vi "SPI Write Read.vi"(5 "CS Pin (10)":u8=10, 7 "SPI Frame Size":u8, 8 "Error In":errorcluster, 9 "Data":u8[](array[numeric]), 10 "SPI Channel (0)":u8, 11 "LINX Resource":T2) -> (0 "Error Out":errorcluster, 1 "Read Data":u8[](array[numeric]), 3 "LINX Resource":T2)   [LabVIEW 2013, in "LVH-LINX.lvlib"]
doc: "Write/Read the specified SPI channel. SPI is full duplex, therefore the write and read operations take place simultaneously."
uses:
  <vilib>/LabVIEW Hacker/LINX/LVH-LINX.lvlib
  <vilib>/LabVIEW Hacker/LINX/Private/Type Defs/LINX Ref.ctl
  <vilib>/LabVIEW Hacker/LINX/Private/Type Defs/Platform.ctl
  <vilib>/LabVIEW Hacker/LINX/Private/Type Defs/Interface.ctl
  <vilib>/LabVIEW Hacker/LINX/Private/Device/Type Defs/LINX Device Config.ctl
  <vilib>/LabVIEW Hacker/LINX/Private/Device/Type Defs/TCP Config.ctl
  <vilib>/LabVIEW Hacker/LINX/Private/Type Defs/Device Family.ctl
  <vilib>/LabVIEW Hacker/LINX/Private/Type Defs/Peripherals/SPI/SPI CS Logic Level.ctl
  <vilib>/LabVIEW Hacker/LINX/Private/Type Defs/Peripheral.ctl
  <vilib>/LabVIEW Hacker/LINX/Private/Type Defs/Channel FGV States.ctl
  <vilib>/LabVIEW Hacker/LINX/Private/Device/Device.lvlib
  <vilib>/myRIO/Common/Instrument Driver Framework/myRIO v1.0/SPI/typedefs/SPI Frame Length.ctl
  <vilib>/myRIO/Common/Instrument Driver Framework/myRIO v1.0/SPI/typedefs/SPI Data Direction.ctl
  <vilib>/myRIO/Common/Instrument Driver Framework/myRIO v1.0/SPI/typedefs/SPI Clock Polarity.ctl
  <vilib>/myRIO/Common/Instrument Driver Framework/myRIO v1.0/SPI/typedefs/SPI Clock Phase.ctl
  <vilib>/myRIO/Instrument Drivers/Onboard IO/SPI/typedefs/SPI Configuration.ctl
  <vilib>/myRIO/Common/Instrument Driver Framework/myRIO v1.0/SPI/typedefs/SPI Channels Enum.ctl
  <vilib>/myRIO/Common/Instrument Driver Framework/Utilities/typedefs/Generic FPGA Reference.ctl
  <vilib>/myRIO/Common/Instrument Driver Framework/Utilities/typedefs/myRIO v1.0 Reference.ctl
  <vilib>/myRIO/Common/Instrument Driver Framework/Utilities/typedefs/Hardware Version Enum.ctl
  <vilib>/myRIO/Common/Instrument Driver Framework/Utilities/typedefs/myRIO Generic Hardware Reference.ctl
  <vilib>/myRIO/Instrument Drivers/Onboard IO/SPI/typedefs/SPI Reference.ctl
panel:
  in  "CS Logic Level":T1
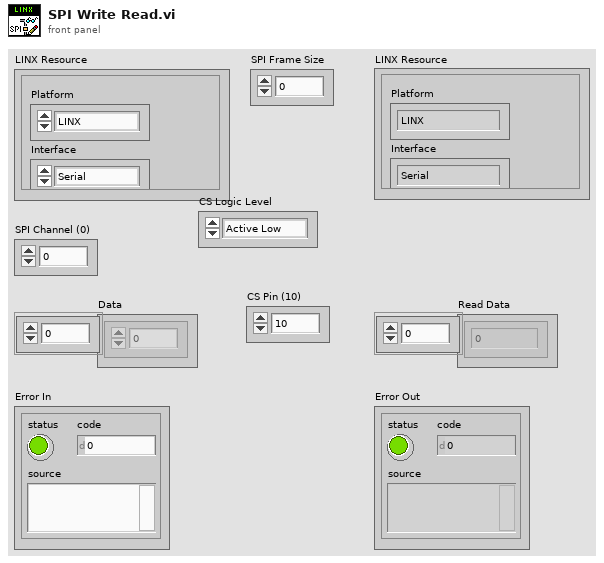
[diagram p1: front panel]
types:
  T1 = typedef "LVH-LINX.lvlib/SPI CS Logic Level.ctl" = enum8{"Active Low", "Active High"}
  T2 = typedef "LVH-LINX.lvlib/LINX Ref.ctl" = cluster{"Platform":T3, "Interface":T4, "LINX Device Config":T5}
  T3 = typedef "LVH-LINX.lvlib/Platform.ctl" = enum16{"LINX", "myRIO"}
  T4 = typedef "LVH-LINX.lvlib/Interface.ctl" = enum16{"Serial", "TCP"}
  T5 = typedef "LVH-LINX.lvlib/Device.lvlib/LINX Device Config.ctl" = cluster{"Interface":T4, "COM Port":refnum<visa-resource-name>, "TCP Configuration":T6, "Device Family":T7, "Device ID":u8, "Device Name":string, "TCP Ref":refnum<k5>}
  T6 = typedef "LVH-LINX.lvlib/Device.lvlib/TCP Config.ctl" = cluster{"IP Address":string, "Port":u16}
  T7 = typedef "LVH-LINX.lvlib/Device Family.ctl" = enum8{"National Instruments", "Digilent", "Arduino"}
  T8 = typedef "LVH-LINX.lvlib/Peripheral.ctl" = enum8{"DI", "DO", "AI", "AO", "PWM", "QE", "UART", "I2C", "SPI", "CAN"}
  T9 = typedef "LVH-LINX.lvlib/Channel FGV States.ctl" = enum16{"Initialize", "Get", "Set"}
  T10 = typedef "SPI.lvlib/SPI Reference.ctl" = cluster{"myRIO Reference":T11, "SPI Channels Enum":T15, "SPI Configuration":T16}
  T11 = typedef "myRIO Generic Hardware Reference.ctl" = cluster{"myRIO Model":T12, "myRIO Hardware Reference":T13}
  T12 = typedef "Hardware Version Enum.ctl" = enum16{"Unknown", "myRIO-1900", "myRIO-1950"}
  T13 = typedef "myRIO v1.0 Reference.ctl" = cluster{"Generic FPGA Reference":T14, "Allow multiple opens":bool}
  T14 = typedef "Generic FPGA Reference.ctl" = refnum<k20>
  T15 = typedef "SPI Channels Enum.ctl" = enum16{"Not Connected", "A/SPI", "B/SPI"}
  T16 = typedef "SPI.lvlib/SPI Configuration.ctl" = cluster{"Frequency (Hz)":dbl, "Clock Phase":T17, "Clock Polarity":T18, "Data Direction":T19, "Frame Length":T20}
  T17 = typedef "SPI Clock Phase.ctl" = enum8{"Leading", "Trailing"}
  T18 = typedef "SPI Clock Polarity.ctl" = enum8{"Low", "High"}
  T19 = typedef "SPI Data Direction.ctl" = enum8{"Most Significant Bit First", "Least Significant Bit First"}
  T20 = typedef "SPI Frame Length.ctl" = u8
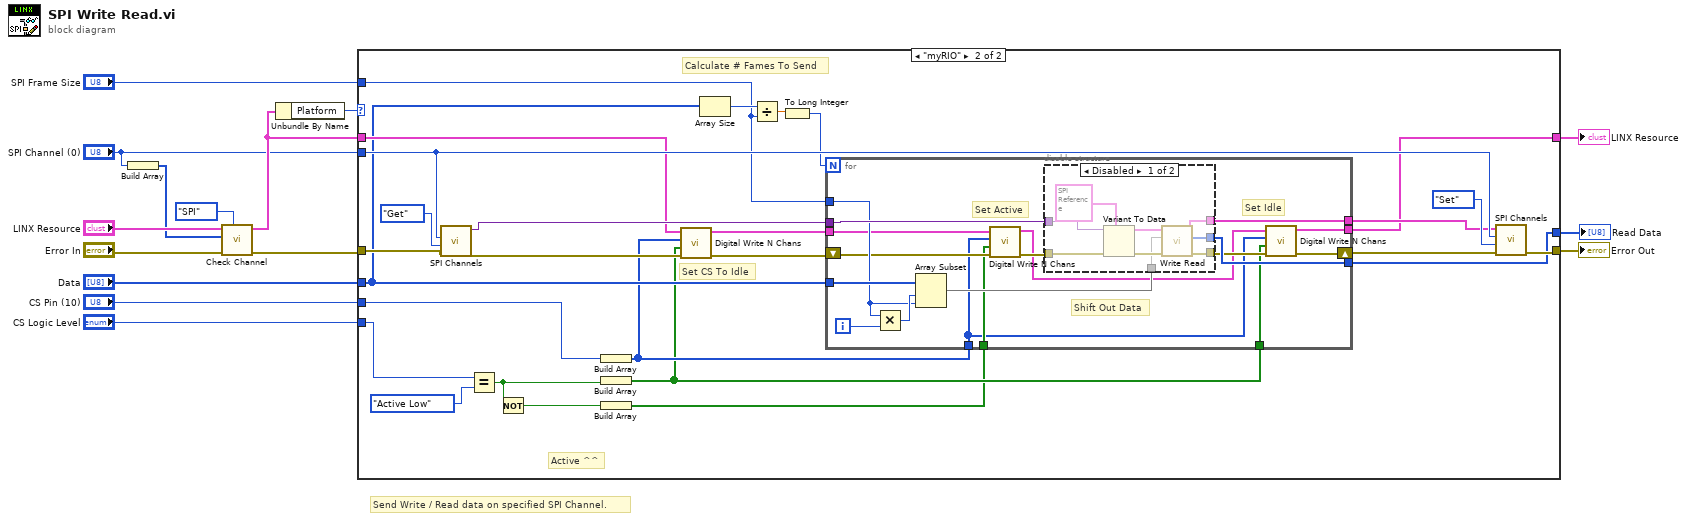
[diagram p0: block diagram]
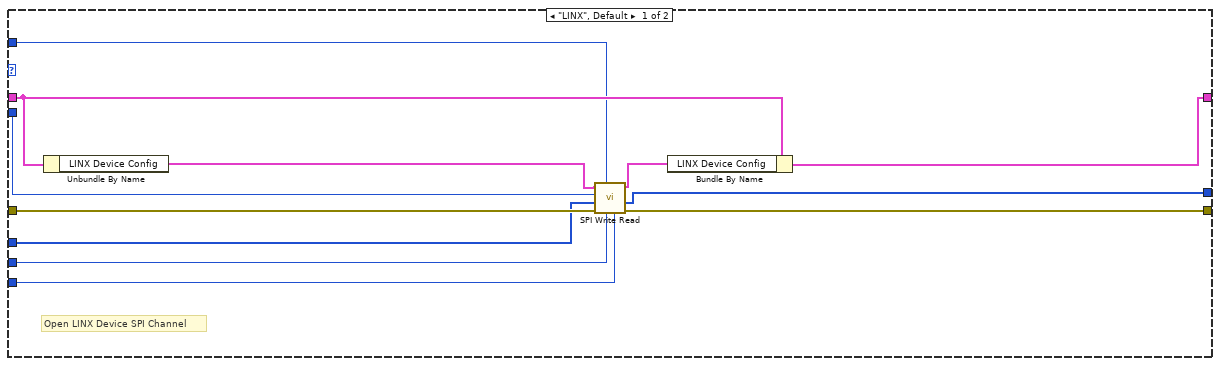
[diagram p2: hidden frame]
diagram:
  # "Send Write / Read data on specified SPI Channel."
  n1 = Build Array("SPI Channel (0)") -> (w9:u8[])
  n2 = call <vilib>:"Check Channel.vi"("Peripheral"=Peripheral."SPI", "Error In"="Error In", "Channels"=w9, "LINX Resource"="LINX Resource") -> ("Error Out"=w10:errorcluster, "LINX Resource"=w11:T2)  [unwired: 5 in, 1 out]
  n3 = Unbundle By Name(w11) -> ("Platform"=w15:T3)
  n4 = case shown="\"myRIO\"" w15 {
    tunnel: w10 -> [w25 w52]
    tunnel: w11 -> [w27 w45]
    tunnel: [w26 w54] -> w14
    tunnel: [w16 w33] -> w1
    tunnel: "SPI Channel (0)" -> [w20 w51]
    tunnel: [w22 w46] -> w6
    tunnel: "Data" -> [w21 w40]
    tunnel: "SPI Frame Size" -> [w19 w36]
    tunnel: "CS Pin (10)" -> [w18 w32]
    tunnel: "CS Logic Level" -> [w17 w42]
    frame "LINX", Default {
      # "Open LINX Device SPI Channel"
      n5 = Unbundle By Name(w27) -> ("LINX Device Config"=w23:T5)
      n6 = call <vilib>:"SPI Write Read.vi"("CS Logic Level"=w17, "CS Pin (10)"=w18, "SPI Frame Size (1)"=w19, "Error In"=w25, "Data"=w21, "SPI Channel"=w20, "LINX Device Config"=w23) -> ("Error Out"=w26:errorcluster, "Read Data"=w22:u8[], "LINX Device Config"=w24:T5)  [unwired: 2 in]
      n7 = Bundle By Name(cluster=w27, "LINX Device Config"=w24) -> (w16:T2)
    }
    frame "myRIO" {
      # "Active ^^"
      # "Calculate # Fames To Send"
      # "Set CS To Idle"
      n8 = call <vilib>:"SPI Channels.vi"("Error In"=w52, "Channel State"=Channel_FGV_States."Get", "Channel Number"=w51) -> ("Error Out"=w44:errorcluster, "SPI Channel"=w47:variant)  [unwired: 7 in]
      n9 = Equal?(x=w42, y=SPI_CS_Logic_Level."Active Low") -> (x = y?=w31:bool)
      n10 = Not(x=w31) -> (.not. x?=w29:bool)
      n11 = Build Array(w32) -> (w34:u8[])
      n12 = Build Array(w31) -> (w30:bool[])
      n13 = Build Array(w29) -> (w28:bool[])
      n14 = call <vilib>:"Digital Write N Chans.vi"("Error In"=w44, "Values"=w30, "DO Channels"=w34, "LINX Resource"=w45) -> ("Error Out"=w43:errorcluster, "LINX Resource"=w35:T2)  [unwired: 6 in]
      n15 = Array Size(array=w40) -> (size(s)=w39:i32)
      n16 = Divide(x=w39, y=w36) -> (x/y=w38:dbl)
      n17 = To Long Integer(number=w38) -> (32bit integer=w37:i32)
      n18 = for {
        N: w37 -> [_]
        tunnel: [w72] -> w48
        tunnel: w47 -> [w71]
        tunnel: w40 -> [w69]
        tunnel: [w70] -> w46
        shift-right: [w61] -> w49
        shift-left: w43 -> [w64]
        tunnel: w36 -> [w65]
        tunnel: w35 -> [w62]
        tunnel: w34 -> [w55]
        tunnel: [w58] -> w33
        tunnel: w30 -> [w57]
        tunnel: w28 -> [w56]
        i -> [w67]
        # "Set Idle"
        # "Shift Out Data"
        # "Set Active"
        n19 = Multiply(x=w65, y=w67) -> (x*y=w66:i32)
        n20 = Array Subset(array=w69, index=w66, length=w65) -> (w68:u8[])
        n21 = call <vilib>:"Digital Write N Chans.vi"("Error In"=w64, "Values"=w56, "DO Channels"=w55, "LINX Resource"=w62) -> ("Error Out"=w63:errorcluster, "LINX Resource"=w59:T2)  [unwired: 6 in]
        n22 = disable-structure shown="Disabled" {
          disable-tunnel: [w79 _] -> w60
          disable-tunnel: w63 -> [w77 _]
          disable-tunnel: [w76 _] -> w72
          disable-tunnel: w71 -> [w75 _]
          disable-tunnel: w68 -> [w74 _]
          disable-tunnel: [w73 _] -> w70
          frame Disabled {
            n23 = Variant To Data(error in=w77, type=T10 {"myRIO Reference"={"myRIO Model"=enum."Unknown", "myRIO Hardware Reference"={"Generic FPGA Reference"=refnum, "Allow multiple opens"=FALSE}}, "SPI Channels Enum"=enum."Not Connected", "SPI Configuration"={"Frequency (Hz)"=0.0, "Clock Phase"=enum."Leading", "Clock Polarity"=enum."Low", "Data Direction"=enum."Most Significant Bit First", "Frame Length"=8}} ("SPI Ref In"), Variant=w75) -> (data=w80:T10, error out=w78:errorcluster)
            n24 = call <vilib>:"Write Read.vi"("error in (no error)"=w78, "Frames to Write"=w74, "SPI Ref In"=w80) -> ("error out"=w79:errorcluster, "Frames Read"=w73:u16[], "SPI Ref Out"=w76:T10)  [unwired: 6 in]
          }
          frame Enabled {
          }
        }
        n25 = call <vilib>:"Digital Write N Chans.vi"("Error In"=w60, "Values"=w57, "DO Channels"=w55, "LINX Resource"=w59) -> ("Error Out"=w61:errorcluster, "LINX Resource"=w58:T2)  [unwired: 6 in]
      }
      n26 = call <vilib>:"SPI Channels.vi"("Error In"=w49, "Channel State"=Channel_FGV_States."Set", "Channel Number"=w51, "SPI Channel"=w48) -> ("Error Out"=w54:errorcluster)  [unwired: 6 in, 1 out]
    }
  }
  "Error Out" <- w14
  "LINX Resource" <- w1
  "Read Data" <- w6
